vi "Compute Path.vi"(11 "AD* in":refnum<class "NI_Robotics_AnytimeDStar.lvclass">) -> (3 "AD* out":refnum<class "NI_Robotics_AnytimeDStar.lvclass">)   [LabVIEW 2017, in "NI_Robotics_AnytimeDStar.lvclass"]
uses:
  <vilib>/robotics/Navigation/Anytime D Star/NI_Robotics_AnytimeDStar.lvclass
  <vilib>/robotics/Navigation/Anytime D Star/NI_Robotics_AnytimeDStar.lvclass/NI_Robotics_AnytimeDStar.ctl
  <vilib>/robotics/Navigation/shared/MapNode/AbstractDstarNode/NI_Robotics_AbstractDstarNode.lvclass
  c:/Program Files (x86)/National Instruments/LabVIEW 2017/vi.lib/robotics/Navigation/shared/MapNode/AbstractMapNode/NI_Robotics_AbstractMapNode.lvclass
  <vilib>/robotics/Navigation/shared/MapNode/AbstractMapNode/NI_Robotics_AbstractMapNode.lvclass
  <vilib>/robotics/Navigation/shared/WorldMap/AbstractDstarWorldMap/NI_Robotics_AbstractDstarWorldMap.lvclass
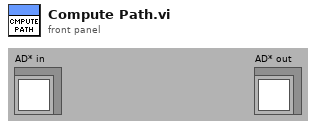
[diagram p1: front panel]
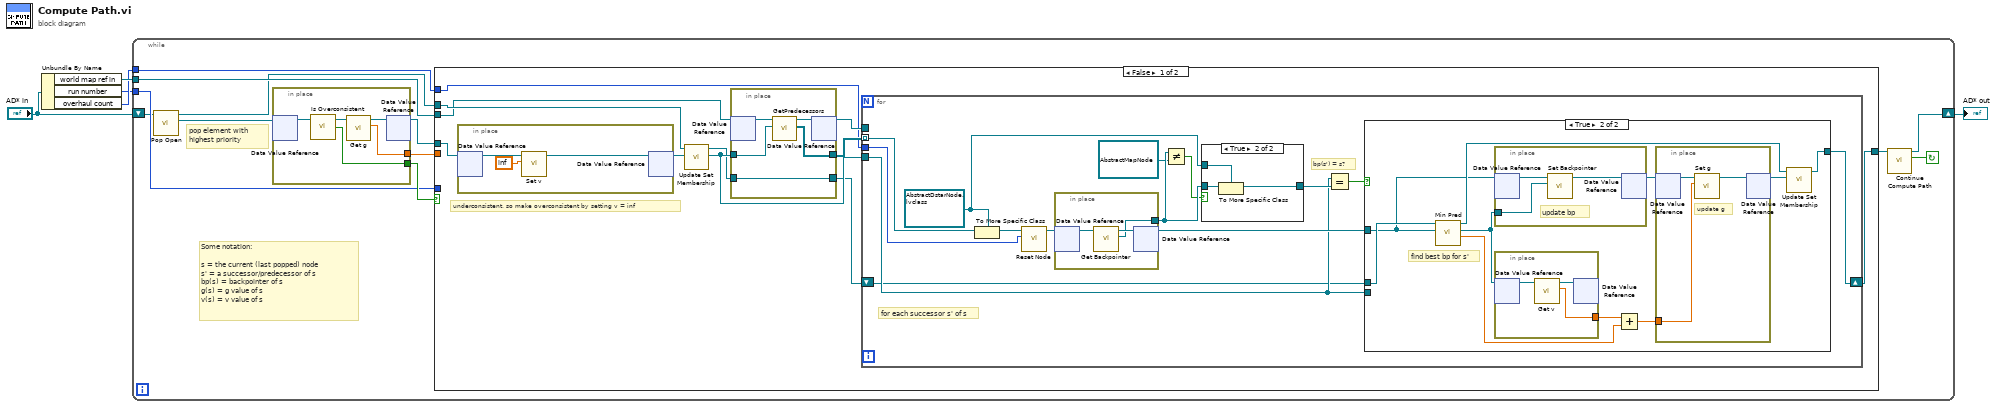
[diagram p0: block diagram]
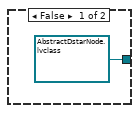
[diagram p2: hidden frame]
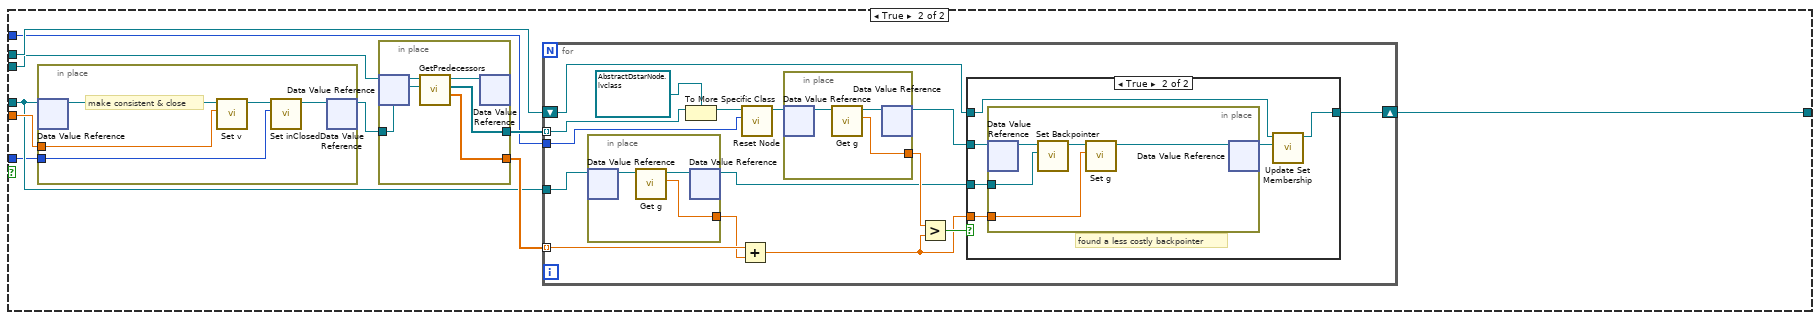
[diagram p4: hidden frame]
diagram:
  n1 = Unbundle By Name("AD* in") -> ("world map ref in"=w5:refnum<data-value>, "run number"=w2:i32, "overhaul count"=w3:i32)
  n2 = while {
    tunnel: w2 -> [w13]
    tunnel: w5 -> [w12]
    shift-right: [w6] -> w4
    shift-left: "AD* in" -> [w9]
    tunnel: w3 -> [w11]
    stop <- w10 continue-if-true
    # "pop element with\nhighest priority"
    # "Some notation:\n\ns = the current (last popped) node\ns' = a successor/predecessor of s\nbp(s) = backpointer of s\ng(s) = g value of s\nv(s) = v value of s"
    n3 = call <vilib>:"Pop Open.vi"("AD* in"=w9) -> ("node ref out"=w14:refnum<data-value>, "AD* out"=w8:refnum<class "NI_Robotics_AnytimeDStar.lvclass">)  [unwired: 8 in, 1 out]
    n4 = in-place {
      in-place-border: [w131] -> w17
      in-place-border: [w135] -> w16
      n5 = in-place-dvr #1(w14) -> (w134:refnum<class "NI_Robotics_AbstractDstarNode.lvclass">)  [unwired: 1 out]
      n6 = call <vilib>:"Is Overconsistent.vi"("AbstractDstarNode in"=w134) -> ("is Overconsistent"=w131:bool, "AbstractDstarNode out"=w133:refnum<class "NI_Robotics_AbstractDstarNode.lvclass">)  [unwired: 2 in, 1 out]
      n7 = call <vilib>:"Get g.vi"("AbstractDstarNode in"=w133) -> ("g"=w135:dbl, "AbstractDstarNode out"=w132:refnum<class "NI_Robotics_AbstractDstarNode.lvclass">)  [unwired: 9 in]
      n8 = in-place-dvr #1(w132) -> (w15:refnum<data-value>)  [unwired: 1 out]
    }
    n9 = case shown="False" w17 {
      tunnel: w16 -> [_ w87]
      tunnel: w13 -> [_ w80]
      tunnel: w15 -> [w28 w83]
      tunnel: w8 -> [w26 w82]
      tunnel: [w18 w81] -> w7
      tunnel: w12 -> [w20 w79]
      tunnel: w11 -> [w19 w78]
      frame False {
        # "underconsistent, so make overconsistent by setting v = inf"
        n10 = in-place {
          n11 = in-place-dvr #2(w28) -> (w76:refnum<class "NI_Robotics_AbstractDstarNode.lvclass">)  [unwired: 1 out]
          n12 = call <vilib>:"Set v.vi"("v"=inf, "AbstractDstarNode in"=w76) -> ("AbstractDstarNode out"=w75:refnum<class "NI_Robotics_AbstractDstarNode.lvclass">)  [unwired: 9 in]
          n13 = in-place-dvr #2(w75) -> (w25:refnum<data-value>)  [unwired: 1 out]
        }
        n14 = call <vilib>:"Update Set Membership.vi"("node ref in"=w25, "AD* in"=w26) -> ("node ref out"=w27:refnum<data-value>, "AD* out"=w22:refnum<class "NI_Robotics_AnytimeDStar.lvclass">)  [unwired: 8 in]
        n15 = in-place {
          in-place-border: w27 -> [w31]
          in-place-border: [w29] -> w24
          in-place-border: w22 -> [w33]
          in-place-border: [w33] -> w21
          n16 = in-place-dvr #3(w20) -> (w32:refnum<class "NI_Robotics_AbstractDstarWorldMap.lvclass">)  [unwired: 1 out]
          n17 = call-dynamic "GetPredecessors.vi"("NodeReference"=w31, "WorldMap in"=w32) -> ("Predecessors"=w29:refnum<data-value>[], "WorldMap out"=w30:refnum<class "NI_Robotics_AbstractDstarWorldMap.lvclass">)  [unwired: 6 in, 2 out]
          n18 = in-place-dvr #3(w30) -> (w23:refnum<data-value>)  [unwired: 1 out]
        }
        n19 = for {
          tunnel: w24 -> [w47] mode=indexing
          tunnel: w27 -> [w42]
          tunnel: w23 -> [_]
          tunnel: w19 -> [w38]
          shift-right: [w34] -> w18
          shift-left: w21 -> [w41]
          w45 = refnum<data-value> refnum ("data value reference")
          # "for each successor s' of s"
          # "bp(s') = s?"
          n20 = To More Specific Class(target class=w45, reference=w47) -> (specific class reference=w40:refnum<data-value>)  [unwired: 1 in, 1 out]
          n21 = call <vilib>:"Reset Node.vi"("overhaul count"=w38, "node reference in"=w40) -> ("node reference out"=w39:refnum<data-value>)  [unwired: 9 in]
          n22 = in-place {
            in-place-border: [w72] -> w37
            n23 = in-place-dvr #4(w39) -> (w74:refnum<class "NI_Robotics_AbstractDstarNode.lvclass">)  [unwired: 1 out]
            n24 = call <vilib>:"Get Backpointer.vi"("AbstractDstarNode in"=w74) -> ("BackPointer"=w72:refnum<data-value>, "AbstractDstarNode out"=w73:refnum<class "NI_Robotics_AbstractDstarNode.lvclass">)  [unwired: 8 in, 1 out]
            n25 = in-place-dvr #4(w73) -> (w43:refnum<data-value>)  [unwired: 1 out]
          }
          n26 = Not Equal?(x=w37, y=refnum<data-value> refnum ("BackPointer")) -> (x != y?=w35:bool)
          n27 = case shown="True" w35 {
            tunnel: [refnum<data-value> refnum ("data value reference") w51] -> w46
            tunnel: w45 -> [_ w50]
            tunnel: w37 -> [_ w49]
            frame False {
            }
            frame True {
              n28 = To More Specific Class(target class=w50, reference=w49) -> (specific class reference=w51:refnum<data-value>)  [unwired: 1 in, 1 out]
            }
          }
          n29 = Equal?(x=w42, y=w46) -> (x = y?=w44:bool)
          n30 = case shown="True" w44 {
            tunnel: w43 -> [_ w55]
            tunnel: w42 -> [_ _]
            tunnel: [w52 w59] -> w34
            tunnel: w41 -> [w52 w57]
            frame False {
              # "g(s') does not depend on s, so do not update"
            }
            frame True {
              # "find best bp for s'"
              n31 = call <vilib>:"Min Pred.vi"("node ref in"=w55, "AD* in"=w57) -> ("cost of node to min pred"=w58:dbl, "min node ref"=w54:refnum<data-value>, "AD* out"=w56:refnum<class "NI_Robotics_AnytimeDStar.lvclass">)  [unwired: 6 in, 1 out]
              n32 = in-place {
                in-place-border: w54 -> [w65]
                # "update bp"
                n33 = in-place-dvr #5(w55) -> (w64:refnum<class "NI_Robotics_AbstractDstarNode.lvclass">)  [unwired: 1 out]
                n34 = call <vilib>:"Set Backpointer.vi"("BackPointer"=w65, "AbstractDstarNode in"=w64) -> ("AbstractDstarNode out"=w63:refnum<class "NI_Robotics_AbstractDstarNode.lvclass">)  [unwired: 8 in, 1 out]
                n35 = in-place-dvr #5(w63) -> (w53:refnum<data-value>)  [unwired: 1 out]
              }
              n36 = in-place {
                in-place-border: [w66] -> w62
                n37 = in-place-dvr #6(w54) -> (w68:refnum<class "NI_Robotics_AbstractDstarNode.lvclass">)  [unwired: 1 out]
                n38 = call <vilib>:"Get v.vi"("AbstractDstarNode in"=w68) -> ("v"=w66:dbl, "AbstractDstarNode out"=w67:refnum<class "NI_Robotics_AbstractDstarNode.lvclass">)  [unwired: 9 in]
                n39 = in-place-dvr #6(w67) -> ()  [unwired: 2 out]
              }
              n40 = Add(x=w62, y=w58) -> (x+y=w61:dbl)
              n41 = in-place {
                in-place-border: w61 -> [w69]
                # "update g"
                n42 = in-place-dvr #7(w53) -> (w71:refnum<class "NI_Robotics_AbstractDstarNode.lvclass">)  [unwired: 1 out]
                n43 = call <vilib>:"Set g.vi"("g"=w69, "AbstractDstarNode in"=w71) -> ("AbstractDstarNode out"=w70:refnum<class "NI_Robotics_AbstractDstarNode.lvclass">)  [unwired: 9 in]
                n44 = in-place-dvr #7(w70) -> (w60:refnum<data-value>)  [unwired: 1 out]
              }
              n45 = call <vilib>:"Update Set Membership.vi"("node ref in"=w60, "AD* in"=w56) -> ("AD* out"=w59:refnum<class "NI_Robotics_AnytimeDStar.lvclass">)  [unwired: 8 in, 1 out]
            }
          }
        }
      }
      frame True {
        n46 = in-place {
          in-place-border: w87 -> [w97]
          in-place-border: w80 -> [w95]
          # "make consistent & close"
          n47 = in-place-dvr #8(w83) -> (w94:refnum<class "NI_Robotics_AbstractDstarNode.lvclass">)  [unwired: 1 out]
          n48 = call <vilib>:"Set v.vi"("v"=w97, "AbstractDstarNode in"=w94) -> ("AbstractDstarNode out"=w96:refnum<class "NI_Robotics_AbstractDstarNode.lvclass">)  [unwired: 9 in]
          n49 = call <vilib>:"Set inClosed.vi"("inClosed"=w95, "AbstractDstarNode in"=w96) -> ("AbstractDstarNode out"=w93:refnum<class "NI_Robotics_AbstractDstarNode.lvclass">)  [unwired: 8 in, 1 out]
          n50 = in-place-dvr #8(w93) -> (w84:refnum<data-value>)  [unwired: 1 out]
        }
        n51 = in-place {
          in-place-border: [w88] -> w86
          in-place-border: [w90] -> w85
          in-place-border: w84 -> [w91]
          n52 = in-place-dvr #9(w79) -> (w92:refnum<class "NI_Robotics_AbstractDstarWorldMap.lvclass">)  [unwired: 1 out]
          n53 = call-dynamic "GetPredecessors.vi"("NodeReference"=w91, "WorldMap in"=w92) -> ("EdgeCost"=w90:dbl[], "Predecessors"=w88:refnum<data-value>[], "WorldMap out"=w89:refnum<class "NI_Robotics_AbstractDstarWorldMap.lvclass">)  [unwired: 6 in, 1 out]
          n54 = in-place-dvr #9(w89) -> ()  [unwired: 2 out]
        }
        n55 = for {
          tunnel: w86 -> [w102] mode=indexing
          tunnel: w85 -> [w104] mode=indexing
          tunnel: w83 -> [w112]
          shift-right: [w105] -> w81
          shift-left: w82 -> [w106]
          tunnel: w78 -> [w100]
          n56 = in-place {
            in-place-border: [w125] -> w103
            n57 = in-place-dvr #10(w112) -> (w127:refnum<class "NI_Robotics_AbstractDstarNode.lvclass">)  [unwired: 1 out]
            n58 = call <vilib>:"Get g.vi"("AbstractDstarNode in"=w127) -> ("g"=w125:dbl, "AbstractDstarNode out"=w126:refnum<class "NI_Robotics_AbstractDstarNode.lvclass">)  [unwired: 9 in]
            n59 = in-place-dvr #10(w126) -> (w108:refnum<data-value>)  [unwired: 1 out]
          }
          n60 = To More Specific Class(target class=refnum<data-value> refnum ("data value reference"), reference=w102) -> (specific class reference=w99:refnum<data-value>)  [unwired: 1 in, 1 out]
          n61 = Add(x=w104, y=w103) -> (x+y=w107:dbl)
          n62 = call <vilib>:"Reset Node.vi"("overhaul count"=w100, "node reference in"=w99) -> ("node reference out"=w98:refnum<data-value>)  [unwired: 9 in]
          n63 = in-place {
            in-place-border: [w128] -> w111
            n64 = in-place-dvr #11(w98) -> (w130:refnum<class "NI_Robotics_AbstractDstarNode.lvclass">)  [unwired: 1 out]
            n65 = call <vilib>:"Get g.vi"("AbstractDstarNode in"=w130) -> ("g"=w128:dbl, "AbstractDstarNode out"=w129:refnum<class "NI_Robotics_AbstractDstarNode.lvclass">)  [unwired: 9 in]
            n66 = in-place-dvr #11(w129) -> (w109:refnum<data-value>)  [unwired: 1 out]
          }
          n67 = Greater?(x=w111, y=w107) -> (0:w110:bool)
          n68 = case shown="True" w110 {
            tunnel: w109 -> [_ w119]
            tunnel: w108 -> [_ w114]
            tunnel: w107 -> [_ w118]
            tunnel: w106 -> [w113 w117]
            tunnel: [w113 w115] -> w105
            frame False {
              # "neighbor's current bp is less costly, so leave alone"
            }
            frame True {
              # "found a less costly backpointer"
              n69 = in-place {
                in-place-border: w114 -> [w123]
                in-place-border: w118 -> [w122]
                n70 = in-place-dvr #12(w119) -> (w124:refnum<class "NI_Robotics_AbstractDstarNode.lvclass">)  [unwired: 1 out]
                n71 = call <vilib>:"Set Backpointer.vi"("BackPointer"=w123, "AbstractDstarNode in"=w124) -> ("AbstractDstarNode out"=w121:refnum<class "NI_Robotics_AbstractDstarNode.lvclass">)  [unwired: 8 in, 1 out]
                n72 = call <vilib>:"Set g.vi"("g"=w122, "AbstractDstarNode in"=w121) -> ("AbstractDstarNode out"=w120:refnum<class "NI_Robotics_AbstractDstarNode.lvclass">)  [unwired: 9 in]
                n73 = in-place-dvr #12(w120) -> (w116:refnum<data-value>)  [unwired: 1 out]
              }
              n74 = call <vilib>:"Update Set Membership.vi"("node ref in"=w116, "AD* in"=w117) -> ("AD* out"=w115:refnum<class "NI_Robotics_AnytimeDStar.lvclass">)  [unwired: 8 in, 1 out]
            }
          }
        }
      }
    }
    n75 = call <vilib>:"Continue Compute Path.vi"("AD* in"=w7) -> ("continue computing path"=w10:bool, "AD* out"=w6:refnum<class "NI_Robotics_AnytimeDStar.lvclass">)  [unwired: 9 in]
  }
  "AD* out" <- w4
